vi "Generador_Funciones.vi"() -> ()   [LabVIEW 2016]
panel:
  out "Waveform Chart":dbl(graph)
  in  "Enum":T1(ring)
  out "Numeric Control":dbl
  in  "Stop Button":bool
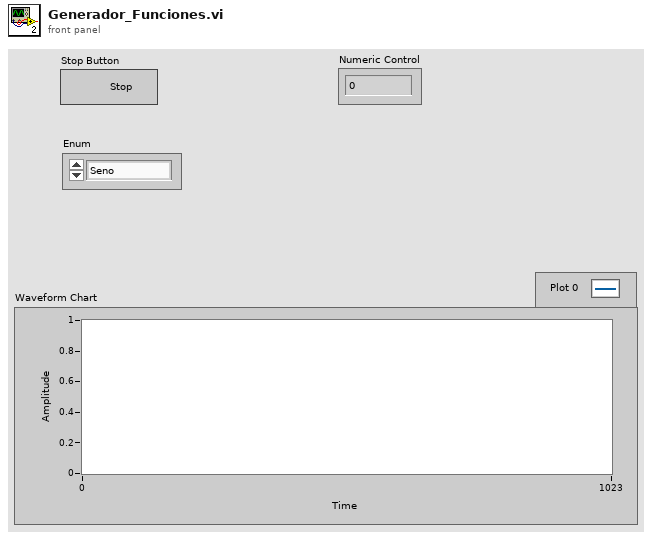
[diagram p1: front panel]
types:
  T1 = enum16{"Seno", "Triangular", "Diente de Sierra", "Pulso", "Secante", "DC", "GND"}
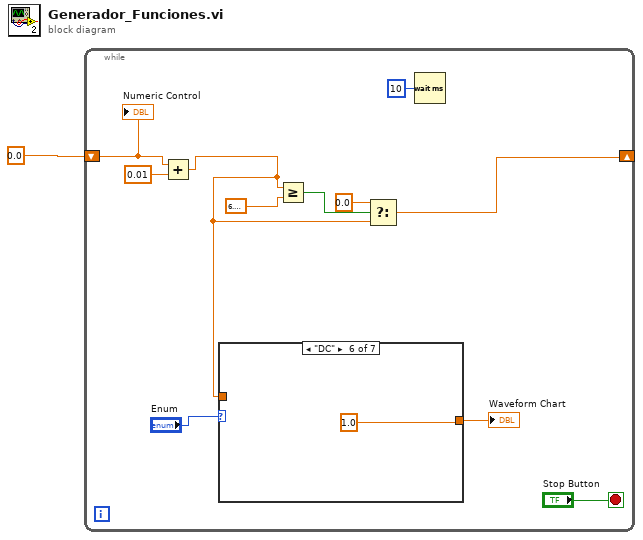
[diagram p0: block diagram]
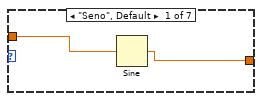
[diagram p2: hidden frame]
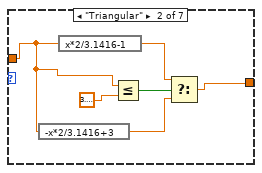
[diagram p3: hidden frame]
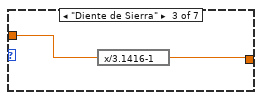
[diagram p4: hidden frame]
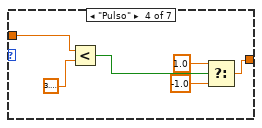
[diagram p5: hidden frame]
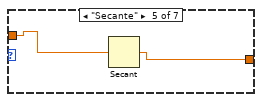
[diagram p6: hidden frame]
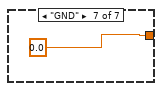
[diagram p7: hidden frame]
diagram:
  n1 = while {
    shift-right: [w5] -> _
    shift-left: 0.0 -> [w12]
    stop <- "Stop Button" stop-if-true
    n2 = Add(x=w12, y=0.01) -> (x+y=w3:dbl)
    n3 = case shown="\"DC\"" "Enum" {
      tunnel: w3 -> [w14 w20 w22 w27 w30 _ _]
      tunnel: [w13 w17 w21 w23 w29 1.0 ("y") 0.0 ("y")] -> w2
      frame "Seno", Default {
        n4 = Sine(x=w14) -> (sin(x)=w13:dbl)
      }
      frame "Triangular" {
        n5 = expression code="-x*2/3.1416+3"(w20) -> (w16:dbl)
        n6 = expression code="x*2/3.1416-1"(w20) -> (w15:dbl)
        n7 = Less Or Equal?(x=w20, y=3.141592653589793) -> (x <= y?=w18:bool)
        n8 = Select(t=w15, s=w18, f=w16) -> (s? t:f=w17:dbl)
      }
      frame "Diente de Sierra" {
        n9 = expression code="x/3.1416-1"(w22) -> (w21:dbl)
      }
      frame "Pulso" {
        n10 = Less?(x=w27, y=3.141592653589793) -> (x < y?=w28:bool)
        n11 = Select(t=1.0, s=w28, f=-1.0) -> (s? t:f=w23:dbl)
      }
      frame "Secante" {
        n12 = Secant(1:w30) -> (0:w29:dbl)
      }
      frame "DC" {
      }
      frame "GND" {
      }
    }
    "Waveform Chart" <- w2
    n13 = Greater Or Equal?(x=w3, y=6.283185307179586) -> (x >= y?=w7:bool)
    n14 = Select(t=0.0, s=w7, f=w3) -> (s? t:f=w5:dbl)
    n15 = Wait (ms)(milliseconds to wait=u32 10) -> ()  [unwired: 1 out]
    "Numeric Control" <- w12
  }
